vi "Is school zone.vi"(8 "error in (no error)":errorcluster, 9 "Current Position":cluster{"X":dbl, "Y":dbl}, 10 "School zone speed":dbl=4.0, 11 "Default speed":dbl=4.0) -> (0 "error out":errorcluster, 3 "Output speed":dbl=50.0)   [LabVIEW 2016]
panel:
  in  "Lower school limit":cluster{"X":dbl, "Y":dbl}={"X"=2090.0, "Y"=2200.0}
  in  "Upper school limit":cluster{"X":dbl, "Y":dbl}={"X"=3990.0, "Y"=4000.0}
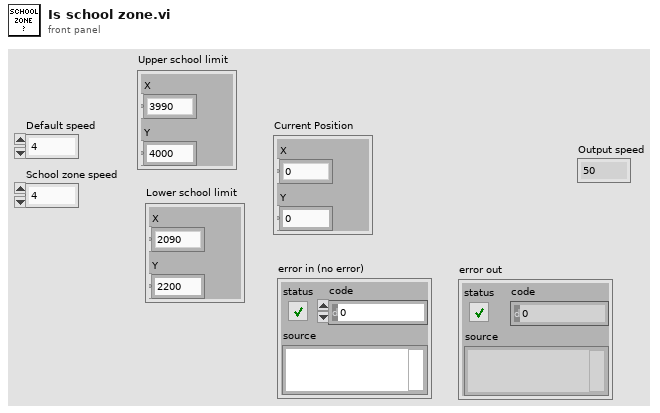
[diagram p1: front panel]
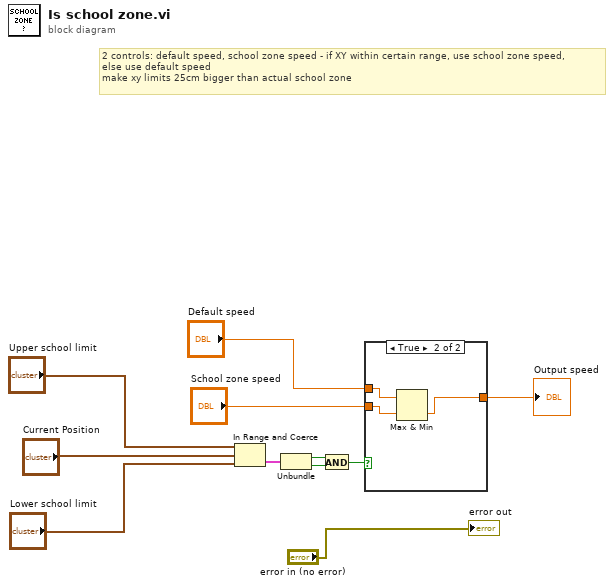
[diagram p0: block diagram]
diagram:
  # "2 controls: default speed, school zone speed - if XY within certain range, use school zone speed,\nelse use default speed\nmake xy limits 25cm bigger than actual school zone"
  n1 = In Range and Coerce(upper limit="Upper school limit", x="Current Position", lower limit="Lower school limit") -> (In Range?=w8:cluster{"X":bool, "Y":bool})  [unwired: 1 out]
  n2 = Unbundle(w8) -> ("X"=w7:bool, "Y"=w6:bool)
  n3 = And(x=w7, y=w6) -> (x .and. y?=w5:bool)
  n4 = case shown="True" w5 {
    tunnel: "School zone speed" -> [_ w15]
    tunnel: [w12 w13] -> w3
    tunnel: "Default speed" -> [w12 w14]
    frame False {
    }
    frame True {
      n5 = Max & Min(x=w14, y=w15) -> (min(x,y)=w13:dbl)  [unwired: 1 out]
    }
  }
  "Output speed" <- w3
  "error out" <- "error in (no error)"
